vi "user maped buttons.vi"(3 "previous button state":u32, 4 "gp button info":T2, 5 "map references":T3) -> (0 "current button state":u32, 1 "mapped gp buttons":T1)   [LabVIEW 2012]
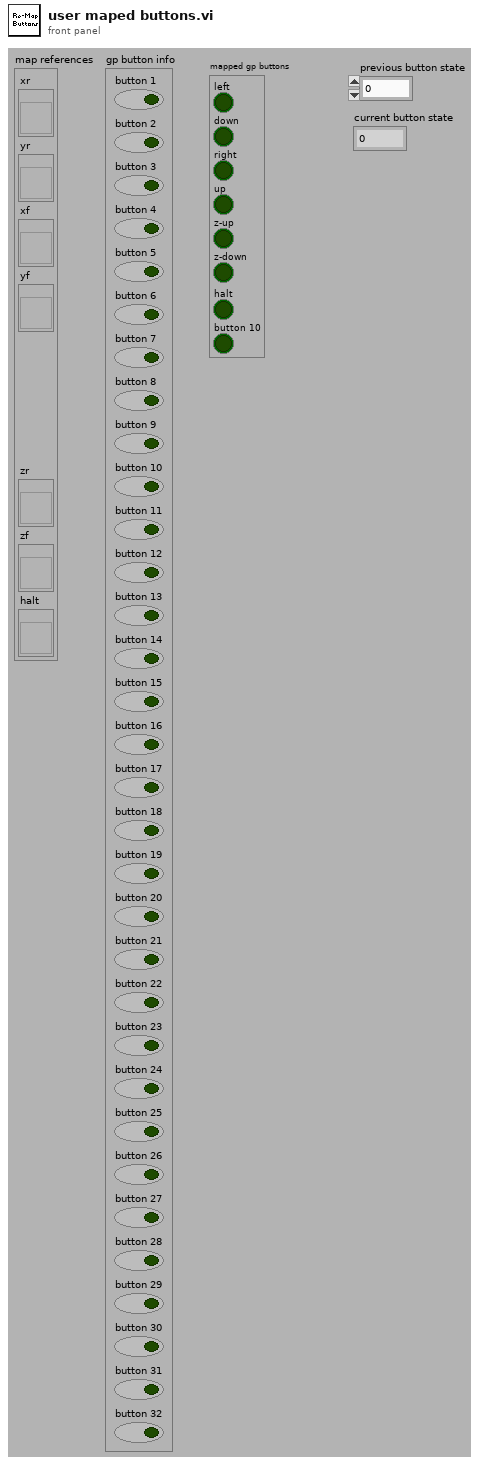
[diagram p1: front panel]
types:
  T1 = cluster{"left":bool, "down":bool, "right":bool, "up":bool, "z-up":bool, "z-down":bool, "halt":bool, "button 10":bool}
  T2 = cluster{"button 1":bool, "button 2":bool, "button 3":bool, "button 4":bool, "button 5":bool, "button 6":bool, "button 7":bool, "button 8":bool, "button 9":bool, "button 10":bool, "button 11":bool, "button 12":bool, "button 13":bool, "button 14":bool, "button 15":bool, "button 16":bool, "button 17":bool, "button 18":bool, "button 19":bool, "button 20":bool, "button 21":bool, "button 22":bool, "button 23":bool, "button 24":bool, "button 25":bool, "button 26":bool, "button 27":bool, "button 28":bool, "button 29":bool, "button 30":bool, "button 31":bool, "button 32":bool}
  T3 = cluster{"xr":refnum<vi>, "yr":refnum<vi>, "xf":refnum<vi>, "yf":refnum<vi>, "zf":refnum<vi>, "zr":refnum<vi>, "halt":refnum<vi>}
  T4 = cluster{"[0]":bool, "[1]":bool, "[2]":bool, "[3]":bool, "[4]":bool, "[5]":bool, "[6]":bool, "[7]":bool, "[8]":bool}
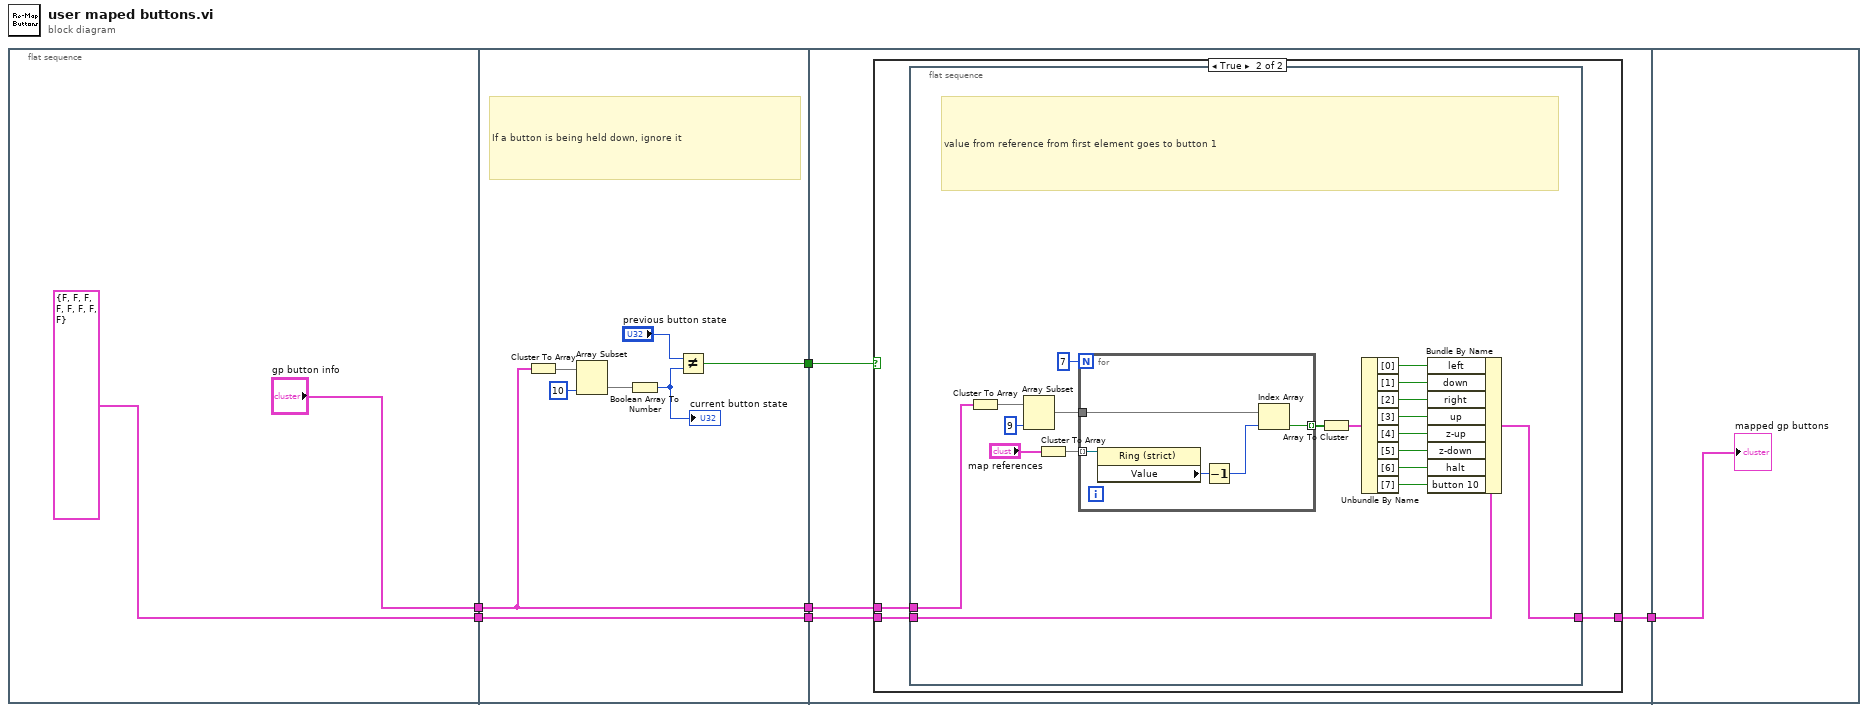
[diagram p0: block diagram]
diagram:
  n1 = flat-sequence {
    tunnel: ["gp button info"] -> w6
    tunnel: [T1 {"left"=FALSE, "down"=FALSE, "right"=FALSE, "up"=FALSE, "z-up"=FALSE, "z-down"=FALSE, "halt"=FALSE, "button 10"=FALSE} ("button info")] -> w2
    tunnel: w6 -> [w10]
    tunnel: [w10] -> w5
    tunnel: [w11] -> w4
    tunnel: [w9] -> w3
    tunnel: w2 -> [w9]
    tunnel: w5 -> [w20]
    tunnel: w4 -> [w19]
    tunnel: w3 -> [w18]
    tunnel: [w17] -> w1
    tunnel: w1 -> [w49]
    frame #0 {
    }
    frame #1 {
      # "If a button is being held down, ignore it"
      n2 = Cluster To Array(cluster=w10) -> (array=w12:bool[])
      n3 = Array Subset(array=w12, length=10) -> (w14:bool[])  [unwired: 1 in]
      n4 = Boolean Array To Number(Boolean array=w14) -> (number=w15:u32)
      "current button state" <- w15
      n5 = Not Equal?(x="previous button state", y=w15) -> (x != y?=w11:bool)
    }
    frame #2 {
      n6 = case shown="True" w19 {
        tunnel: w20 -> [_ w24]
        tunnel: w18 -> [w21 w23]
        tunnel: [w21 w22] -> w17
        frame False {
        }
        frame True {
          n7 = flat-sequence {
            tunnel: [w42] -> w22
            tunnel: w23 -> [w43]
            tunnel: w24 -> [w33]
            frame #0 {
              # "value from reference from first element goes to button 1"
              n8 = Cluster To Array(cluster=w33) -> (array=w39:bool[])
              n9 = Array Subset(array=w39, length=9) -> (w38:bool[])  [unwired: 1 in]
              n10 = Cluster To Array(cluster="map references") -> (array=w34:refnum<vi>[])
              n11 = for {
                N: 7 -> [_]
                tunnel: w34 -> [w48] mode=indexing
                tunnel: w38 -> [w47]
                tunnel: [w44] -> w37 mode=indexing
                n12 = property on="Property Node" class="Ring (strict)"(reference=w48) -> ("Value"=w46:u16)  [unwired: 1 in, 2 out]
                n13 = Decrement(x=w46) -> (x-1=w45:u16)
                n14 = Index Array(array=w47, index=w45) -> (element=w44:bool)
              }
              n15 = Array To Cluster(array=w37) -> (cluster=w41:T4)
              n16 = Unbundle By Name(w41) -> ("[0]"=w32:bool, "[1]"=w31:bool, "[2]"=w30:bool, "[3]"=w29:bool, "[4]"=w28:bool, "[5]"=w27:bool, "[6]"=w26:bool, "[7]"=w25:bool)
              n17 = Bundle By Name(cluster=w43, "left"=w32, "down"=w31, "right"=w30, "up"=w29, "z-up"=w28, "z-down"=w27, "halt"=w26, "button 10"=w25) -> (w42:T1)
            }
          }
        }
      }
    }
    frame #3 {
      "mapped gp buttons" <- w49
    }
  }
